vi "Move To Impl.vi"(8 "error in (no error)":errorcluster, 9 "Index":u16, 10 "Area":enum16{"Home", "Well", "Wash Port"}(ring), 11 "Alltesta Autosampler in":refnum<class "Alltesta Autosampler.lvclass">) -> (0 "error out":errorcluster, 3 "Alltesta Autosampler out":refnum<class "Alltesta Autosampler.lvclass">)   [LabVIEW 2023, in "Alltesta Autosampler.lvlib" / "Alltesta Autosampler.lvclass"]
uses:
  Alltesta Autosampler.lvclass
  Alltesta Autosampler.lvclass/Alltesta Autosampler.ctl
  Alltesta Autosampler.lvlib
panel:
  out "raw response":string
  out "Parsed Response":string
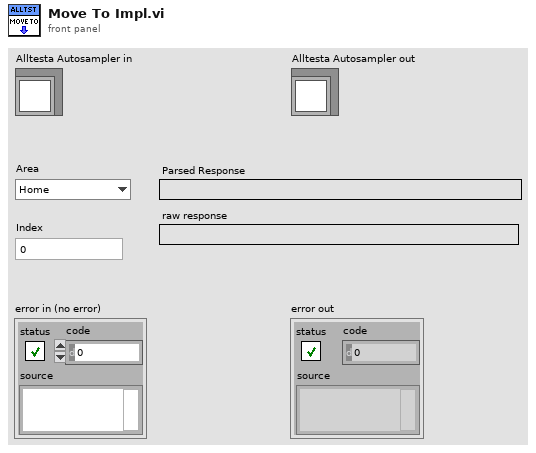
[diagram p1: front panel]
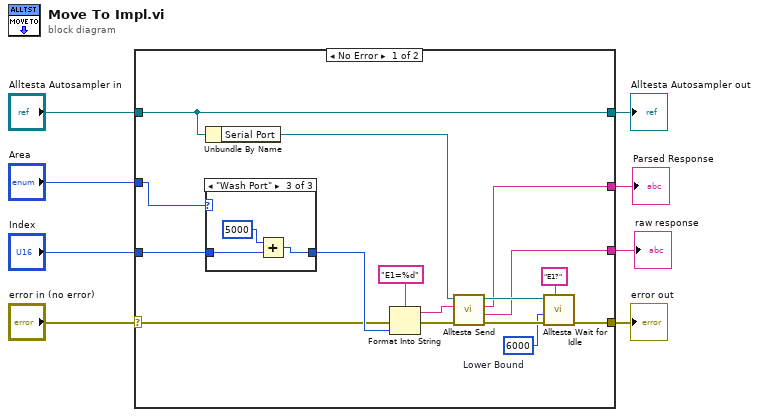
[diagram p0: block diagram]
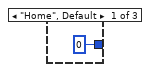
[diagram p2: hidden frame]
diagram:
  n1 = case shown="No Error" "error in (no error)" {
    selector: "error in (no error)" -> [w18 w31]
    tunnel: [w11 w31] -> w7
    tunnel: "Alltesta Autosampler in" -> [w17 w30]
    tunnel: [w17 w30] -> w5
    tunnel: "Area" -> [w21 _]
    tunnel: "Index" -> [w20 _]
    tunnel: [w10 _] -> w2
    tunnel: [w9 _] -> w1
    frame No Error {
      w12 = 6000  # Lower Bound
      n2 = Unbundle By Name(w17) -> ("Serial Port"=w16:refnum<visa-resource-name>)
      n3 = case shown="\"Wash Port\"" w21 {
        tunnel: w20 -> [_ w26 w29]
        tunnel: [u16 0 ("Index") w26 w28] -> w19
        frame "Home", Default {
        }
        frame "Well" {
        }
        frame "Wash Port" {
          n4 = Add(x=u16 5000, y=w29) -> (x+y=w28:u16)
        }
      }
      n5 = Format Into String(format string="E1=%d", error in=w18, w19) -> (resulting string=w23:string, error out=w24:errorcluster)  [unwired: 1 in]
      n6 = call "Alltesta Send.vi"("error in (no error)"=w24, "Command"=w23, "Serial Port in"=w16) -> ("error out"=w15:errorcluster, "raw response"=w9:string, "Response"=w10:string, "Serial Port out"=w14:refnum<visa-resource-name>)  [unwired: 5 in]
      n7 = call "Alltesta Wait for Idle.vi"("Poll Command"="E1?", "error in (no error)"=w15, "Lower Bound"=w12, "Serial Port in"=w14) -> ("error out"=w11:errorcluster)  [unwired: 6 in, 1 out]
    }
    frame Error {
    }
  }
  "error out" <- w7
  "Alltesta Autosampler out" <- w5
  "Parsed Response" <- w2
  "raw response" <- w1
